vi "Profile Loop to Main.vi"(0 "Current Step":u8, 1 "Step Time Left":u32, 8 "Write (F)":bool) -> (14 "Current Step OUT":u8, 15 "Step Time Left OUT":u32)   [LabVIEW 2019]
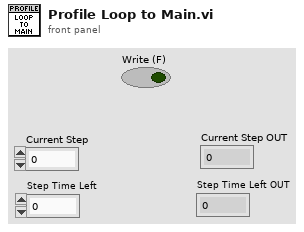
[diagram p1: front panel]
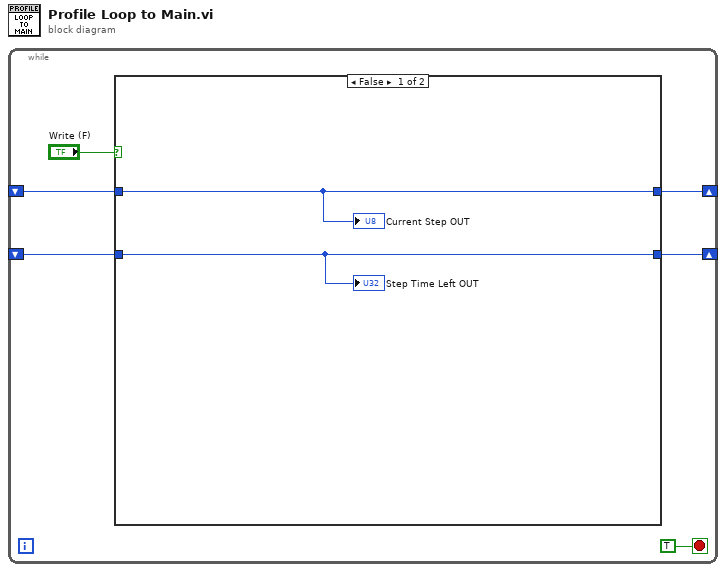
[diagram p0: block diagram]
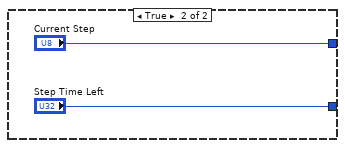
[diagram p2: hidden frame]
diagram:
  n1 = while {
    shift-right: [w4] -> _
    shift-left: _ -> [w2]
    shift-right: [w3] -> _
    shift-left: _ -> [w1]
    stop <- TRUE stop-if-true
    n2 = case shown="False" "Write (F)" {
      tunnel: [w8 "Current Step"] -> w4
      tunnel: [w7 "Step Time Left"] -> w3
      tunnel: w2 -> [w8 _]
      tunnel: w1 -> [w7 _]
      frame False {
        "Current Step OUT" <- w8
        "Step Time Left OUT" <- w7
      }
      frame True {
      }
    }
  }
